vi "Get_operation_mode.vi"(8 "error in (no error)":errorcluster, 11 "Connection in":T1={"Baud"=9600, "Flow Ctl"=0, "COM port"="", "Parity"=0} {"Parity" items=["None", "Odd", "Even"]; "Flow Ctl" items=["None"]; "Baud" items=["4800"=4800, "9600"=9600, "19200"=19200, "38400"=38400]}) -> (0 "error out":errorcluster, 1 "CV":bool, 2 "CC":bool, 3 "Connection out":T1={"Baud"=9600, "Flow Ctl"=0, "COM port"="", "Parity"=0} {"Parity" items=["None", "Odd", "Even"]; "Flow Ctl" items=["None"]; "Baud" items=["4800"=4800, "9600"=9600, "19200"=19200, "38400"=38400]})   [LabVIEW 2014, in "B&K Precision 9120 series.lvclass"]
uses:
  B&K Precision 9120 series.lvclass
  Serial_Config.ctl
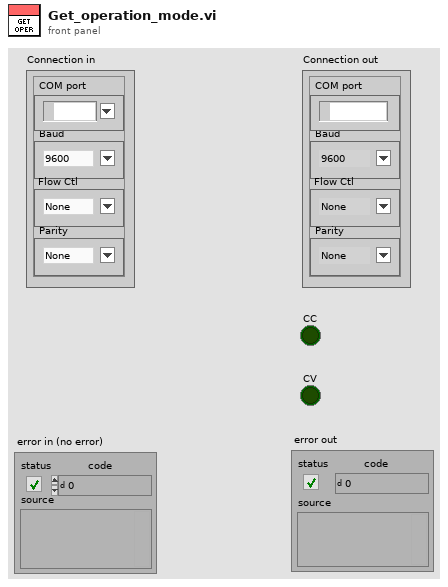
[diagram p1: front panel]
types:
  T1 = typedef "B&K Precision 9120 series.lvclass/Serial_Config.ctl" = cluster{"Baud":u32, "Flow Ctl":u16, "COM port":refnum<visa-resource-name>, "Parity":u16}
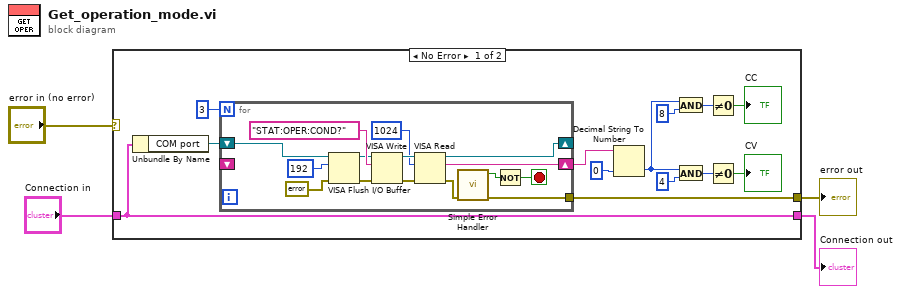
[diagram p0: block diagram]
diagram:
  n1 = case shown="No Error" "error in (no error)" {
    selector: "error in (no error)" -> [_ w34]
    tunnel: "Connection in" -> [w6 w33]
    tunnel: [w6 w33] -> w3
    tunnel: [w5 w34] -> w2
    frame No Error {
      n2 = Unbundle By Name(w6) -> ("COM port"=w7:refnum<visa-resource-name>)
      n3 = for {
        N: 3 -> [_]
        shift-right: [w30] -> _
        shift-left: w7 -> [w22]
        shift-right: [w28] -> w17
        shift-left: _ -> [_]
        tunnel: [w27] -> w5
        stop <- w23 stop-if-true
        n4 = VISA Flush I/O Buffer(VISA resource name=w22, mask (16)=u16 192, error in (no error)=errorcluster {"status"=FALSE, "code"=0, "source"=""} ("error constant")) -> (VISA resource name out=w21:refnum<visa-resource-name>, error out=w19:errorcluster)
        n5 = VISA Write(VISA resource name=w21, write buffer="STAT:OPER:COND?", error in (no error)=w19) -> (VISA resource name out=w32:refnum<visa-resource-name>, error out=w26:errorcluster)  [unwired: 1 out]
        n6 = VISA Read(VISA resource name=w32, byte count=u32 1024, error in (no error)=w26) -> (VISA resource name out=w30:refnum<visa-resource-name>, read buffer=w28:string, error out=w25:errorcluster)  [unwired: 1 out]
        n7 = call <vilib>:"Simple Error Handler.vi"("error in (no error)"=w25) -> ("error?"=w24:bool, "error out"=w27:errorcluster)  [unwired: 4 in, 3 out]
        n8 = Not(x=w24) -> (.not. x?=w23:bool)
      }
      n9 = Decimal String To Number(string=w17, default (0L)=u32 0 ("default (0 DBL)")) -> (number=w13:u32)  [unwired: 1 in, 1 out]
      n10 = And(x=w13, y=u32 8) -> (x .and. y?=w15:u32)
      n11 = And(x=w13, y=u32 4) -> (x .and. y?=w12:u32)
      n12 = Not Equal To 0?(x=w15) -> (x != 0?=→"CC":bool)
      n13 = Not Equal To 0?(x=w12) -> (x != 0?=→"CV":bool)
    }
    frame Error {
    }
  }
  "Connection out" <- w3
  "error out" <- w2
